vi "CRYSet Window Language.vi"(10 "sID":string) -> (1 "sMultibyte_Out":string, 2 "sID_Out":string, 3 "sUnicode_Out":string)   [LabVIEW 2013]
uses:
  CRYMainGlobal.vi
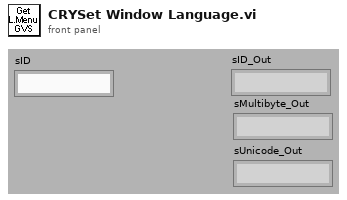
[diagram p1: front panel]
types:
  T1 = enum32{"English", "Chinese", "Korean", "Japanese", "Russian", "Chinese traditional"}
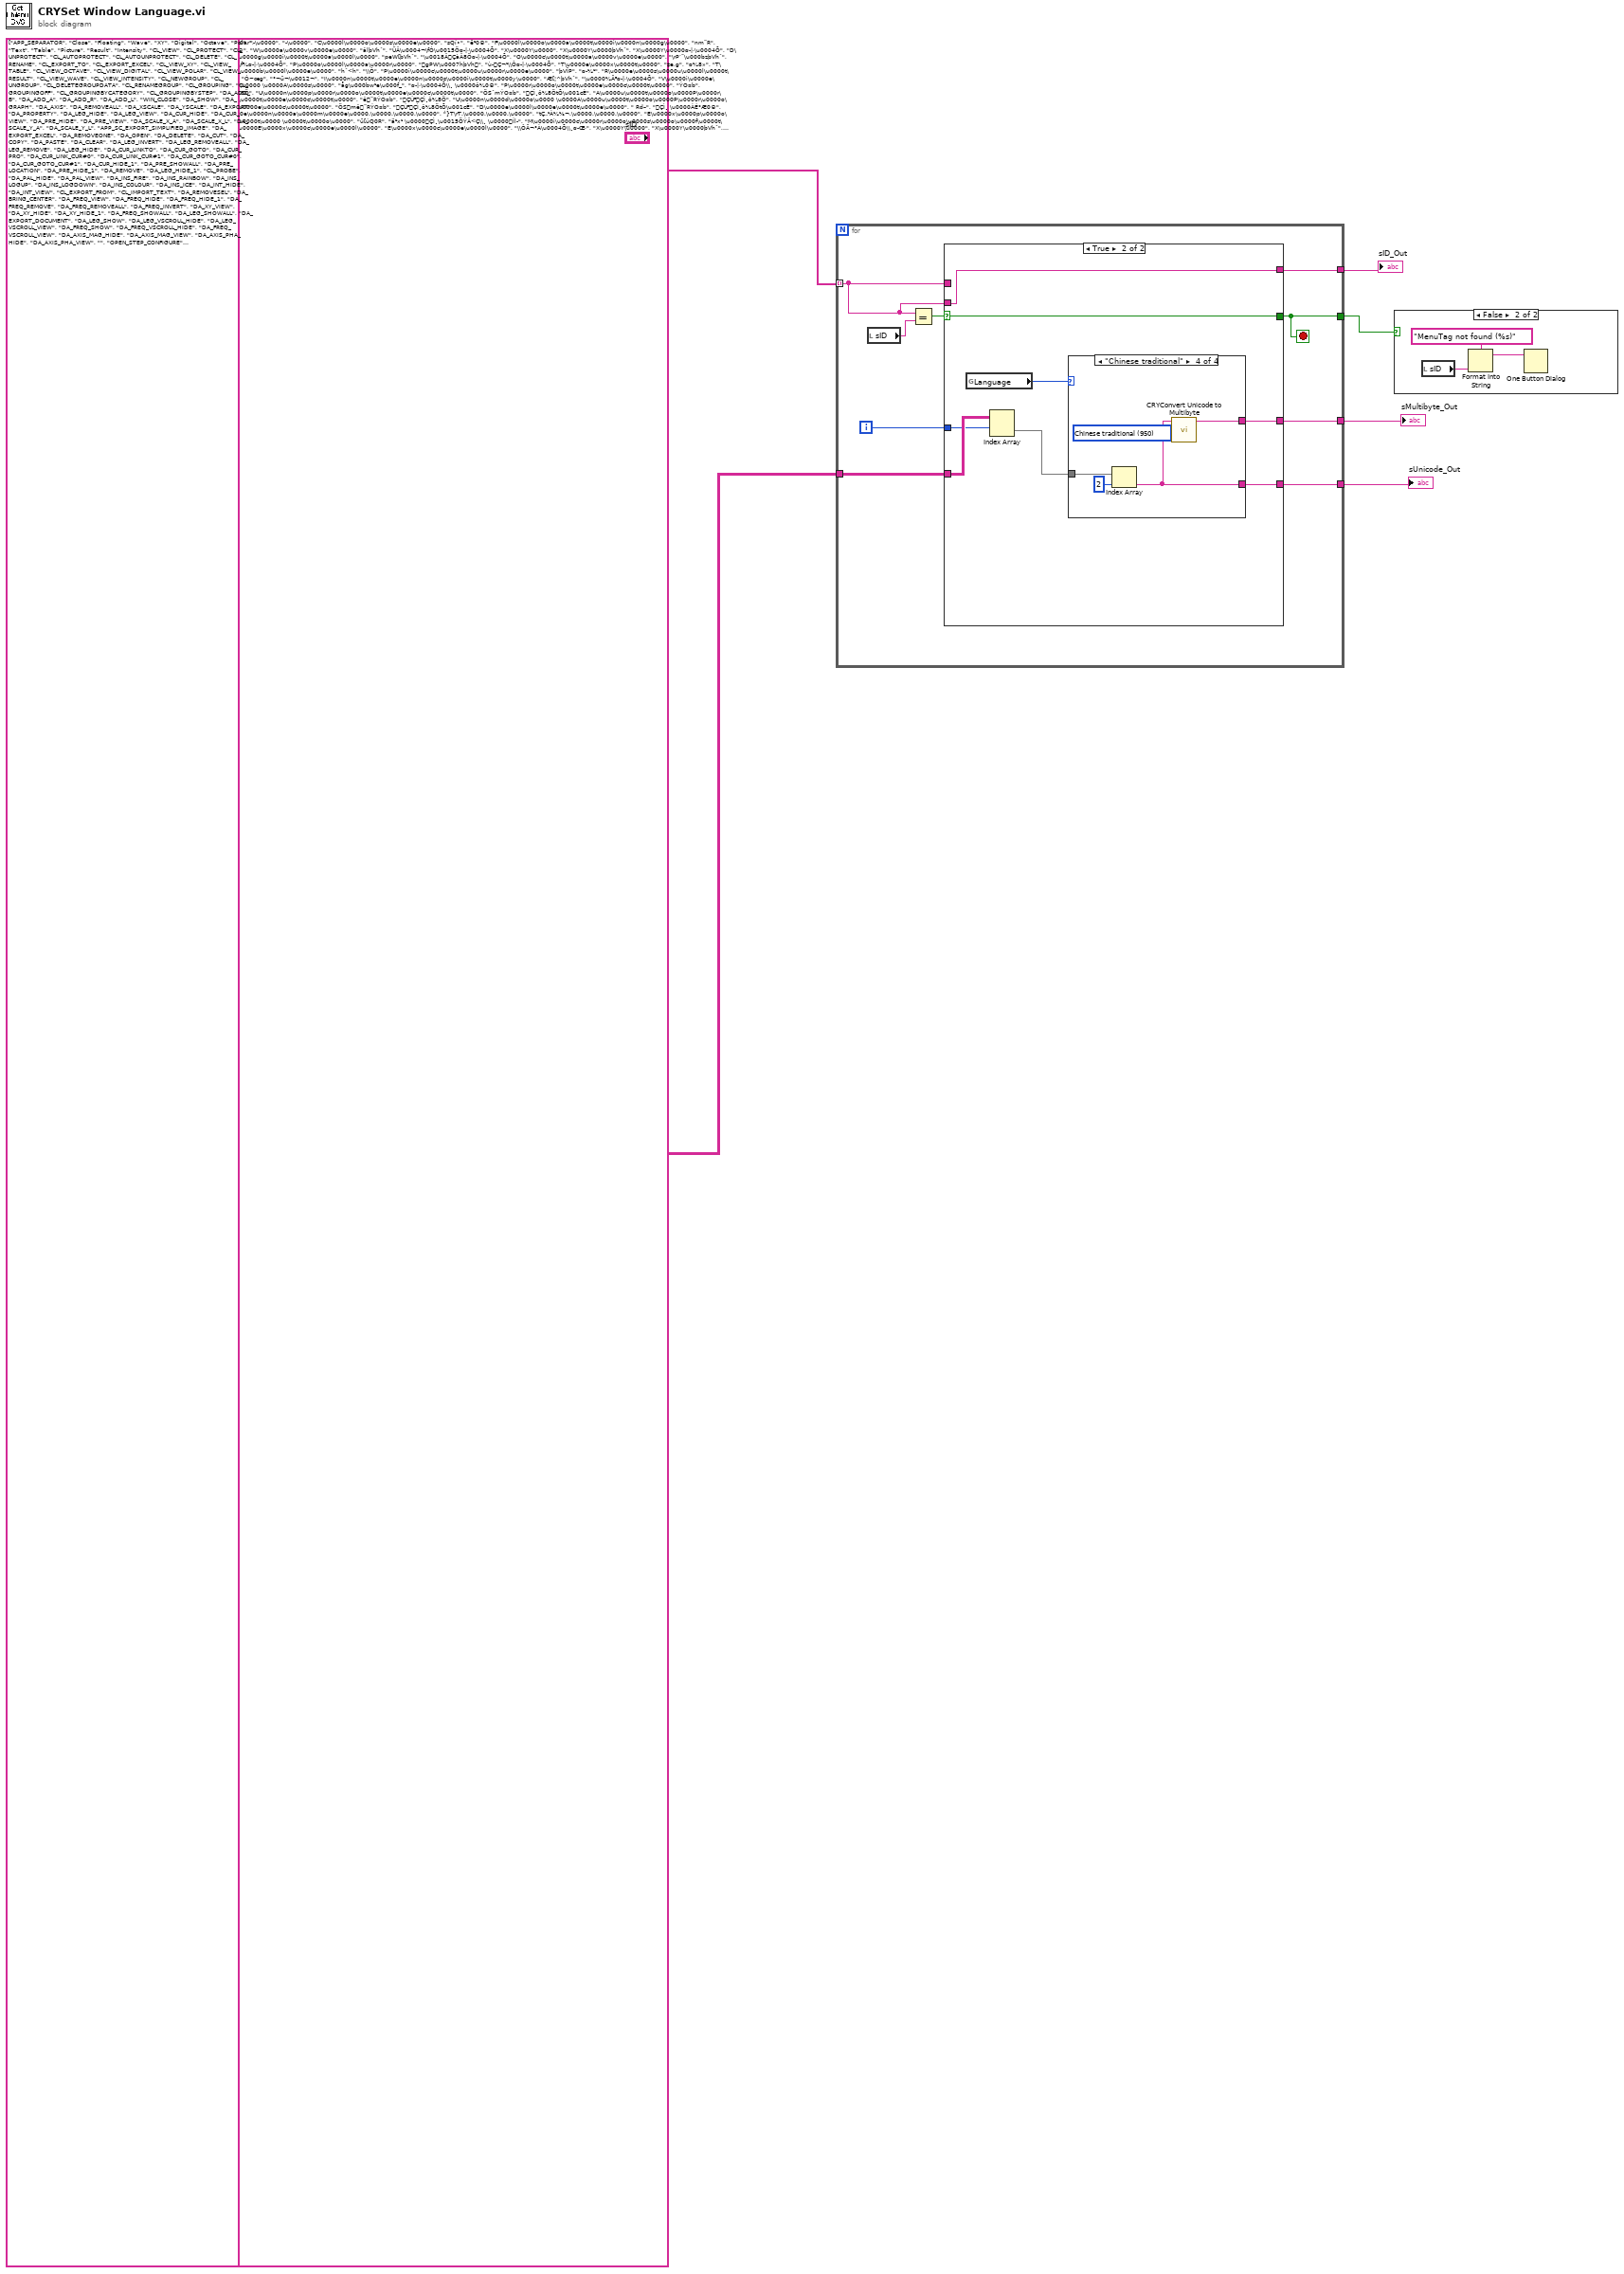
[diagram p0: block diagram]
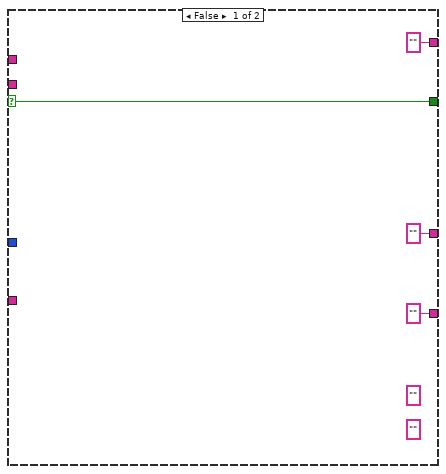
[diagram p3: hidden frame]
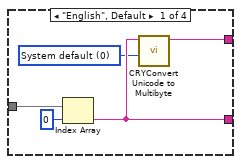
[diagram p4: hidden frame]
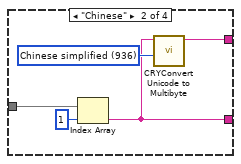
[diagram p5: hidden frame]
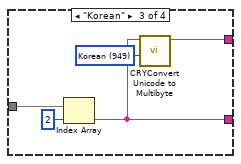
[diagram p6: hidden frame]
diagram:
  # "ASCIICODE"
  # "UNICODE"
  n1 = for {
    tunnel: string[][] [["-\u0000", "-\u0000", "-\u0000"], ["C\u0000l\u0000o\u0000s\u0000e\u0000", "sQí•", "ë²0®"], ["F\u0000l\u0000o\u0000a\u0000t\u0000i\u0000n\u0000g\u0000", "nm¨R", "D·°Æ0®"], ["W\u0000a\u0000v\u0000e\u0000", "âlþVhˆ", "ÜÂ\u0004¬\fÓ\u0015Öø­|·\u0004Õ"], ["X\u0000Y\u0000", "X\u0000Y\u0000þVhˆ", "X\u0000Y\u0000ø­|·\u0004Õ"], ["D\u0000i\u0000g\u0000i\u0000t\u0000a\u0000l\u0000", "peW[þVhˆ", "\u0018ÂÇàÂ8Öø­|·\u0004Õ"], ["O\u0000c\u0000t\u0000a\u0000v\u0000e\u0000", "\rP‘˜\u000bzþVhˆ", "%ÆÀÐ\f¾ø­|·\u0004Õ"], ["P\u0000o\u0000l\u0000a\u0000r\u0000", "gPW\u0007hþVh", "ù­Ç¬¹\\Ôø­|·\u0004Õ"], ["T\u0000e\u0000x\u0000t\u0000", "‡e,g", "ø¼8»"], ["T\u0000a\u0000b\u0000l\u0000e\u0000", "hˆ<h", "\\Ô"], ["P\u0000i\u0000c\u0000t\u0000u\u0000r\u0000e\u0000", "þVÏP", "ø­¼¹"], ["R\u0000e\u0000s\u0000u\u0000l\u0000t\u0000", "Ó~œg", "°¬ü¬\u0012¬"], ["I\u0000n\u0000t\u0000e\u0000n\u0000s\u0000i\u0000t\u0000y\u0000", "Æ[¦^þVhˆ", "\u0000¼Ä³ø­|·\u0004Õ"], ["V\u0000i\u0000e\u0000w\u0000 \u0000A\u0000s\u0000", "åg\u000bw¹e\u000f_", "ø­|·\u0004Õ\\¸ \u0000ô¼0®"], ["P\u0000r\u0000o\u0000t\u0000e\u0000c\u0000t\u0000", "ÝO¤b", "ÇÌ¸ô¼8Ö"], ["U\u0000n\u0000p\u0000r\u0000o\u0000t\u0000e\u0000c\u0000t\u0000", "ÖSˆmÝO¤b", "ÇÌ¸ô¼8ÖtÕ\u001cÈ"], ["A\u0000u\u0000t\u0000o\u0000P\u0000r\u0000o\u0000t\u0000e\u0000c\u0000t\u0000", "ê¨RÝO¤b", "ÇÙ³ÇÌ¸ô¼8Ö"], ["U\u0000n\u0000d\u0000o\u0000 \u0000A\u0000u\u0000t\u0000o\u0000P\u0000r\u0000o\u0000t\u0000e\u0000c\u0000t\u0000", "ÖSmê¨RÝO¤b", "ÇÙ³ÇÌ¸ô¼8ÖtÕ\u001cÈ"], ["D\u0000e\u0000l\u0000e\u0000t\u0000e\u0000", " Rd–", "ÇÌ¸ \u0000ÀÉ°Æ0®"], ["R\u0000e\u0000n\u0000a\u0000m\u0000e\u0000.\u0000.\u0000.\u0000", "͑}T\rT.\u0000.\u0000.\u0000", "tÇ„¹À¼½¬.\u0000.\u0000.\u0000"], ["E\u0000x\u0000p\u0000o\u0000r\u0000t\u0000 \u0000t\u0000o\u0000", "ü[úQ0R", "ä²x¹ \u0000ÇÌ¸\u0015ÖÝÂ<Ç\\¸ \u0000Íl­"], ["M\u0000i\u0000c\u0000r\u0000o\u0000s\u0000o\u0000f\u0000t\u0000 \u0000E\u0000x\u0000c\u0000e\u0000l\u0000", "E\u0000x\u0000c\u0000e\u0000l\u0000", "\\ÔÄ¬°À\u0004Õ\\¸ø­Œ·"], ["X\u0000Y\u0000", "X\u0000Y\u0000þVhˆ", "X\u0000Y\u0000ø­|·\u0004Õ"], ["T\u0000a\u0000b\u0000l\u0000e\u0000", "hˆ<h", "\\Ô=Ì8»"], ["O\u0000c\u0000t\u0000a\u0000v\u0000e\u0000", "\rP‘˜\u000bzþVhˆ", "%ÆÀÐ\f¾ø­|·\u0004Õ"], ["D\u0000i\u0000g\u0000i\u0000t\u0000a\u0000l\u0000", "peW[þVhˆ", "\u0018ÂÇàÂ8Öø­|·\u0004Õ"], ["P\u0000o\u0000l\u0000a\u0000r\u0000", "gPW\u0007hþVh", "ù­Ç¬¹\\Ôø­|·\u0004Õ"], ["R\u0000e\u0000s\u0000u\u0000l\u0000t\u0000", "Ó~œg", "°¬ü¬=Ì8»"], ["W\u0000a\u0000v\u0000e\u0000", "âlþVhˆ", "ÜÂ\u0004¬\fÓ\u0015Öø­|·\u0004Õ"], ["I\u0000n\u0000t\u0000e\u0000n\u0000s\u0000i\u0000t\u0000y\u0000", "Æ[¦^þVhˆ", "\u0000¼Ä³ø­|·\u0004Õ"], ["N\u0000e\u0000w\u0000 \u0000G\u0000r\u0000o\u0000u\u0000p\u0000", "°eú^\u0006RÄ~", "ÈÀø­ù¸"], ["U\u0000n\u0000g\u0000r\u0000o\u0000u\u0000p\u0000", "ÖSˆm\u0006RÄ~", "ø­ù¸tÕ\u001cÈ"], ["D\u0000e\u0000l\u0000e\u0000t\u0000e\u0000 \u0000G\u0000r\u0000o\u0000u\u0000p\u0000 \u0000a\u0000n\u0000d\u0000 \u0000D\u0000a\u0000t\u0000a\u0000", " Rd–\u0006RÄ~penc", "ø­ù¸ \u0000\u000f¼ \u0000ÇÌ¸ÀÉ°Æ0® \u0000"], ["R\u0000e\u0000n\u0000a\u0000m\u0000e\u0000.\u0000.\u0000.\u0000", "͑}T\rT.\u0000.\u0000.\u0000", "tÇ„¹À¼½¬.\u0000.\u0000.\u0000"], ["A\u0000u\u0000t\u0000o\u0000G\u0000r\u0000o\u0000u\u0000p\u0000i\u0000n\u0000g\u0000", "ê¨R\u0006RÄ~", "ø­ù¸TÖ"], ["A\u0000u\u0000t\u0000o\u0000G\u0000r\u0000o\u0000u\u0000p\u0000i\u0000n\u0000g\u0000 \u0000O\u0000f\u0000f\u0000", "sQíê¨R\u0006RÄ~", "ÇÙ³ø­ù¸TÖD°0®"], ["A\u0000u\u0000t\u0000o\u0000G\u0000r\u0000o\u0000u\u0000p\u0000i\u0000n\u0000g\u0000 \u0000b\u0000y\u0000 \u0000C\u0000a\u0000t\u0000e\u0000g\u0000o\u0000r\u0000y\u0000", "\tcgq{|Wê¨R\u0006RÄ~", "½X¹ÐÅ \u0000XÇ\\Õ \u0000ÇÙ³ø­ù¸TÖ"], ["A\u0000u\u0000t\u0000o\u0000G\u0000r\u0000o\u0000u\u0000p\u0000i\u0000n\u0000g\u0000 \u0000b\u0000y\u0000 \u0000S\u0000t\u0000e\u0000p\u0000", "\tcgqek¤ê¨R\u0006RÄ~", "mÕ©ºÐÅ \u0000XÇ\\Õ \u0000ÇÙ³ø­ù¸TÖ"], ["A\u0000d\u0000d\u0000 \u0000B\u0000e\u0000l\u0000o\u0000w\u0000", "\u0011T\u000bNûm R", "DÅ˜·ÐÅ \u0000½À…Ç"], ["A\u0000d\u0000d\u0000 \u0000A\u0000b\u0000o\u0000v\u0000e\u0000", "\u0011T\nNûm R", "捌信 \u0000嚼吳"], ["A\u0000d\u0000d\u0000 \u0000R\u0000i\u0000g\u0000h\u0000t\u0000", "\u0011TóSûm R", "$Æx¹½ÊÐÅ \u0000½À…Ç"], ["A\u0000d\u0000d\u0000 \u0000L\u0000e\u0000f\u0000t\u0000", "\u0011Tæ]ûm R", "|Æ½ÊÐÅ \u0000½À…Ç"], ["R\u0000e\u0000m\u0000o\u0000v\u0000e\u0000", " Rd–", "ë²0®"], ["S\u0000h\u0000o\u0000w\u0000", ">f:y", "\\ÔÜÂ"], ["G\u0000r\u0000a\u0000p\u0000h\u0000 \u0000V\u0000i\u0000e\u0000w\u0000", "ûm RþVhˆ", "ø­|·\u0004Õ \u0000”Í\u0000¬"], ["A\u0000x\u0000i\u0000s\u0000", "E^¦^/\u0000øvMO", "•Í"], ["R\u0000e\u0000m\u0000o\u0000v\u0000e\u0000 \u0000A\u0000l\u0000l\u0000", " Rd–@b\tgòf¿~", "¨ºà´ \u0000ÇÌ¸ÀÉ°Æ0®"], ["X\u0000 \u0000S\u0000c\u0000a\u0000l\u0000e\u0000", "X\u0000 \u0000\u0007h:\\", "X\u0000™ÌÄ³"], ["Y\u0000 \u0000S\u0000c\u0000a\u0000l\u0000e\u0000", "Y\u0000 \u0000\u0007h:\\", "Y\u0000™ÌÄ³"], ["E\u0000x\u0000p\u0000o\u0000r\u0000t\u0000 \u0000t\u0000o\u0000", "ü[úQ0R", "ä²x¹ \u0000ÇÌ¸\u0015ÖÝÂ<Ç\\¸ \u0000Íl­"], ["P\u0000r\u0000o\u0000p\u0000e\u0000r\u0000t\u0000i\u0000e\u0000s\u0000.\u0000.\u0000.\u0000", "^\\'`.\u0000.\u0000.\u0000", "Á1Á.\u0000.\u0000.\u0000"], ["L\u0000e\u0000g\u0000e\u0000n\u0000d\u0000", "þV‹O", "tÇ„¹©º]¸"], ["L\u0000e\u0000g\u0000e\u0000n\u0000d\u0000", "þV‹O", "tÇ„¹©º]¸"], ["C\u0000u\u0000r\u0000s\u0000o\u0000r\u0000", "8n\u0007h", " Ç\\Ô"], ["C\u0000u\u0000r\u0000s\u0000o\u0000r\u0000", "8n\u0007h", " Ç\\Ô"], ["P\u0000r\u0000e\u0000v\u0000i\u0000e\u0000w\u0000", "„˜È‰", "ø»¬¹ô¼0®"], ["P\u0000r\u0000e\u0000v\u0000i\u0000e\u0000w\u0000", "„˜È‰", "ø»¬¹ô¼0®"], ["A\u0000u\u0000t\u0000o\u0000 \u0000S\u0000c\u0000a\u0000l\u0000e\u0000", "ꁨR)>e", "ÇÙ³ÌÄ³"], ["L\u0000o\u0000g\u0000a\u0000r\u0000i\u0000t\u0000h\u0000m\u0000i\u0000c\u0000", "ù[pe", "\\¸ø­™ÌÄ³"], ["A\u0000u\u0000t\u0000o\u0000 \u0000S\u0000c\u0000a\u0000l\u0000e\u0000", "ꁨR)>e", "ÇÙ³ÌÄ³"], ["L\u0000o\u0000g\u0000a\u0000r\u0000i\u0000t\u0000h\u0000m\u0000i\u0000c\u0000", "ù[pe", "\\¸ø­™ÌÄ³"], ["S\u0000i\u0000m\u0000p\u0000l\u0000i\u0000f\u0000i\u0000e\u0000d\u0000 \u0000I\u0000m\u0000a\u0000g\u0000e\u0000", "€{\u0016S„vþVÏP", "\u0004¬è²\\Õ \u0000TÖÁÀ"], ["M\u0000i\u0000c\u0000r\u0000o\u0000s\u0000o\u0000f\u0000t\u0000 \u0000E\u0000x\u0000c\u0000e\u0000l\u0000", "E\u0000x\u0000c\u0000e\u0000l\u0000", "\\ÔÄ¬°À\u0004Õ\\¸ø­Œ·"], ["R\u0000e\u0000m\u0000o\u0000v\u0000e\u0000", " Rd–", "\\Õ\u001c¬ \u0000ÇÌ¸ÀÉ°Æ0®"], ["O\u0000p\u0000e\u0000n\u0000", "Sb\u0000_", "ôÅ0®"], ["D\u0000e\u0000l\u0000e\u0000t\u0000e\u0000", " Rd–", "ÀÉ°Æ0®"], ["C\u0000u\u0000t\u0000", "jR4", "Çt¹0®"], ["C\u0000o\u0000p\u0000y\u0000", "\rY6R", "õ¼¬À"], ["P\u0000a\u0000s\u0000t\u0000e\u0000", "4\nN", "™½tÇ0®"], ["C\u0000l\u0000e\u0000a\u0000r\u0000", "\u0005nd–", "ÀÉ°Æ0®"], ["I\u0000n\u0000v\u0000e\u0000r\u0000t\u0000", "ÍS\t", "\u0018¼\u0004È"], ["R\u0000e\u0000m\u0000o\u0000v\u0000e\u0000 \u0000A\u0000l\u0000l\u0000", " Rd–@b\tg", "¨ºà´ \u0000ÇÌ¸ÀÉ°Æ0®"], ["R\u0000e\u0000m\u0000o\u0000v\u0000e\u0000", " Rd–", "\\Õ\u001c¬ \u0000ÇÌ¸ÀÉ°Æ0®"], ["H\u0000i\u0000d\u0000e\u0000 \u0000L\u0000e\u0000g\u0000e\u0000n\u0000d\u0000", "ÏþVO", "á¬ ÁtÇ„¹ \u0000(Â0®0®"], ["L\u0000i\u0000n\u0000k\u0000 \u0000T\u0000o\u0000 \u0000P\u0000l\u0000o\u0000t\u0000", "þ”¥cØ~6R", "ø­|·\u0004ÕÐÅ \u0000(¸°¬"], ["G\u0000o\u0000 \u0000T\u0000o\u0000 \u0000C\u0000u\u0000r\u0000s\u0000o\u0000r\u0000", "l0R8n\u0007h", " Ç\\Ô\u0004ÇXÎ\\¸ \u0000.Æ0®0®"], ["C\u0000u\u0000r\u0000s\u0000o\u0000r\u0000 \u0000P\u0000r\u0000o\u0000p\u0000e\u0000r\u0000t\u0000i\u0000e\u0000s\u0000.\u0000.\u0000.\u0000", "8n\u0007h„v^\\'`.\u0000.\u0000.\u0000", " Ç\\ÔÁ1Á"], ["C\u0000u\u0000r\u0000s\u0000o\u0000r\u0000 \u00000\u0000", "8n\u0007h0\u0000", " Ç\\Ô \u00000\u0000"], ["C\u0000u\u0000r\u0000s\u0000o\u0000r\u0000 \u00001\u0000", "8n\u0007h1\u0000", " Ç\\Ô \u00001\u0000"], ["C\u0000u\u0000r\u0000s\u0000o\u0000r\u0000 \u00000\u0000", "8n\u0007h0\u0000", " Ç\\Ô \u00000\u0000"], ["C\u0000u\u0000r\u0000s\u0000o\u0000r\u0000 \u00001\u0000", "8n\u0007h1\u0000", " Ç\\Ô \u00001\u0000"], ["H\u0000i\u0000d\u0000e\u0000 \u0000C\u0000u\u0000r\u0000s\u0000o\u0000r\u0000", "Ï8n\u0007h", " Ç\\Ô(Â0®0®"], ["S\u0000h\u0000o\u0000w\u0000 \u0000A\u0000l\u0000l\u0000", ">f:y@b\tg", "\u0004È´Ìô¼ìÅüÈ0®"], ["G\u0000o\u0000 \u0000T\u0000o\u0000 \u0000L\u0000o\u0000c\u0000a\u0000t\u0000i\u0000o\u0000n\u0000", "»SMOn", "\u0004Ö¬Ç\u0004ÇXÎô¼ìÅüÈ0®"], ["H\u0000i\u0000d\u0000e\u0000 \u0000P\u0000r\u0000e\u0000v\u0000i\u0000e\u0000w\u0000", "ÏÈ", "ø»¬¹ô¼0®(Â0®0®"], ["R\u0000e\u0000m\u0000o\u0000v\u0000e\u0000", " Rd–", "ÇÌ¸ÀÉ°Æ0®"], ["H\u0000i\u0000d\u0000e\u0000 \u0000L\u0000e\u0000g\u0000e\u0000n\u0000d\u0000", "ÏÈ", "tÇ„¹©º]¸ \u0000(Â0®0®"], ["S\u0000h\u0000o\u0000w\u0000 \u0000P\u0000r\u0000o\u0000b\u0000e\u0000\u0000", ">f:y¢cˆ”", "\u0000³íÅô¼0®"], ["P\u0000a\u0000l\u0000e\u0000t\u0000t\u0000e\u0000", "þVb_å]wQ", "pÈ…È\u0010Ó"], ["P\u0000a\u0000l\u0000e\u0000t\u0000t\u0000e\u0000", "þVb_å]wQ", "pÈ…È\u0010Ó"], ["F\u0000i\u0000r\u0000e\u0000", "kp\n\u0000\u0000\u0000\n\u0000", "ˆ½8®"], ["R\u0000a\u0000i\u0000n\u0000b\u0000o\u0000w\u0000", "i_y†", "4»ÀÉ\u001c¬"], ["L\u0000o\u0000g\u0000 \u0000u\u0000p\u0000", "ù[pe\nN", "ÃÆ \u0000\\¸ø­"], ["L\u0000o\u0000g\u0000 \u0000d\u0000o\u0000w\u0000n\u0000", "ù[pe\u000bN", "DÅ˜· \u0000\\¸ø­"], ["C\u0000o\u0000l\u0000o\u0000u\u0000r\u0000", "i_r‚", "ÉÀ\b¬"], ["I\u0000c\u0000e\u0000", "°Q", "¼ÅLÇ"], ["I\u0000n\u0000t\u0000e\u0000n\u0000s\u0000i\u0000t\u0000y\u0000", "Æ[¦^þVhˆ", "\u0000¼Ä³ø­|·\u0004Õ"], ["I\u0000n\u0000t\u0000e\u0000n\u0000s\u0000i\u0000t\u0000y\u0000", "Æ[¦^þVhˆ", "\u0000¼Ä³ø­|·\u0004Õ"], ["I\u0000m\u0000p\u0000o\u0000r\u0000t\u0000 \u0000f\u0000o\u0000r\u0000m\u0000", "ÎN‡eöNü[eQ", "\fÓ|Ç\\¸€½0Ñ \u0000…Çl­"], ["T\u0000e\u0000x\u0000t\u0000 \u0000f\u0000i\u0000l\u0000e\u0000", "‡e,g‡eöN", "ø¼8»\fÓ|Ç"], ["R\u0000e\u0000m\u0000o\u0000v\u0000e\u0000 \u0000S\u0000e\u0000l\u0000e\u0000c\u0000t\u0000e\u0000d\u0000 \u0000R\u0000o\u0000w\u0000s\u0000", " Rd\t[vL", " ÁÝÐ\u001c´ \u0000ÕÇÌ¸ÀÉ°Æ0®"], ["B\u0000r\u0000i\u0000n\u0000g\u0000 \u0000t\u0000o\u0000 \u0000C\u0000e\u0000n\u0000t\u0000e\u0000r\u0000", "&^eg„v-Nô•", "\u0011ÉìÂ<Ç\\¸ \u0000tÇÙ³"], ["F\u0000r\u0000e\u0000q\u0000u\u0000e\u0000n\u0000c\u0000y\u0000", "‘˜‡s", "üÈ\fÓ\u0018Â"], ["F\u0000r\u0000e\u0000q\u0000u\u0000e\u0000n\u0000c\u0000y\u0000", "‘˜‡s", "üÈ\fÓ\u0018Â"], ["H\u0000i\u0000d\u0000e\u0000 \u0000F\u0000r\u0000e\u0000q\u0000u\u0000e\u0000n\u0000c\u0000y\u0000", "Ïs", "üÈ\fÓ\u0018Â(Â0®0®"], ["R\u0000e\u0000m\u0000o\u0000v\u0000e\u0000", " Rd–", "\\Õ\u001c¬ \u0000üÈ\fÓ\u0018ÂÀÉ°Æ0®"], ["R\u0000e\u0000m\u0000o\u0000v\u0000e\u0000 \u0000A\u0000l\u0000l\u0000", " Rd–@b\tg", "¨ºà´ \u0000üÈ\fÓ\u0018ÂÀÉ°Æ0®"], ["I\u0000n\u0000v\u0000e\u0000r\u0000t\u0000", "\u0012Pn", "\u0018¼\u0004È"], ["X\u0000Y\u0000 \u0000G\u0000r\u0000a\u0000p\u0000h\u0000", "X\u0000Y\u0000þVhˆ", "X\u0000Y\u0000ø­|·\u0004Õ"], ["X\u0000Y\u0000 \u0000G\u0000r\u0000a\u0000p\u0000h\u0000", "X\u0000Y\u0000þVhˆ", "X\u0000Y\u0000ø­|·\u0004Õ"], ["H\u0000i\u0000d\u0000e\u0000 \u0000X\u0000Y\u0000 \u0000G\u0000r\u0000a\u0000p\u0000h\u0000", "ÏX\u0000Y\u0000þVh", "X\u0000Y\u0000ø­|·\u0004Õ \u0000(Â0®0®"], ["S\u0000h\u0000o\u0000w\u0000 \u0000A\u0000l\u0000l\u0000", ">f:y@b\tg‘˜‡s", "¨ºà´ \u0000 \u0000üÈ\fÓ\u0018Âô¼ìÅüÈ0®"], ["S\u0000h\u0000o\u0000w\u0000 \u0000A\u0000l\u0000l\u0000", ">f:y@b\tg", "¨ºà´ \u0000 \u0000ÇÌ¸ô¼ìÅüÈ0®"], ["D\u0000o\u0000c\u0000u\u0000m\u0000e\u0000n\u0000t\u0000", "‡e,g", "8»\u001cÁ¸ÓÑÉ=Ì8»"], ["S\u0000h\u0000o\u0000w\u0000", ">f:y", "\\ÔÜÂ"], ["V\u0000e\u0000r\u0000t\u0000i\u0000c\u0000a\u0000l\u0000 \u0000S\u0000c\u0000r\u0000o\u0000l\u0000l\u0000b\u0000a\u0000r\u0000", "‚WôvÚn¨Rag", "\u0018ÂÁÉtÇÙ³`·"], ["V\u0000e\u0000r\u0000t\u0000i\u0000c\u0000a\u0000l\u0000 \u0000S\u0000c\u0000r\u0000o\u0000l\u0000l\u0000b\u0000a\u0000r\u0000", "‚WôvÚn¨Rag", "\u0018ÂÁÉtÇÙ³`·"], ["S\u0000h\u0000o\u0000w\u0000", ">f:y", "\\ÔÜÂ"], ["V\u0000e\u0000r\u0000t\u0000i\u0000c\u0000a\u0000l\u0000 \u0000S\u0000c\u0000r\u0000o\u0000l\u0000l\u0000b\u0000a\u0000r\u0000", "‚WôvÚn¨Rag", "\u0018ÂÁÉtÇÙ³`·"], ["V\u0000e\u0000r\u0000t\u0000i\u0000c\u0000a\u0000l\u0000 \u0000S\u0000c\u0000r\u0000o\u0000l\u0000l\u0000b\u0000a\u0000r\u0000", "‚WôvÚn¨Rag", "\u0018ÂÁÉtÇÙ³`·"], ["M\u0000a\u0000g\u0000n\u0000i\u0000t\u0000u\u0000d\u0000e\u0000", "E^¦^", "ÄÉíÓ"], ["M\u0000a\u0000g\u0000n\u0000i\u0000t\u0000u\u0000d\u0000e\u0000", "E^¦^", "ÄÉíÓ"], ["P\u0000h\u0000a\u0000s\u0000e\u0000", "øvMO", "\u0004ÇÁÀ"], ["P\u0000h\u0000a\u0000s\u0000e\u0000", "øvMO", "\u0004ÇÁÀ"], ["", "", ""], ["C\u0000o\u0000n\u0000f\u0000i\u0000g\u0000u\u0000r\u0000e\u0000 \u0000S\u0000t\u0000e\u0000p\u0000.\u0000.\u0000.\u0000", "ek¤šÓ~„g.\u0000.\u0000.\u0000", "¸ÓÑÉ0®l­1Á.\u0000.\u0000.\u0000"], ["M\u0000o\u0000v\u0000e\u0000 \u0000D\u0000o\u0000w\u0000n\u0000", "\u0011T\u000bN\n\u0000\u0000\u0000", "DÅ˜·\\¸ \u0000tÇÙ³"], ["M\u0000o\u0000v\u0000e\u0000 \u0000U\u0000p\u0000", "\u0011T\nN", "°Æ\\¸ \u0000tÇÙ³"], ["D\u0000e\u0000l\u0000e\u0000t\u0000e\u0000", " Rd–", "­À\u001cÈ"], ["C\u0000o\u0000n\u0000f\u0000i\u0000g\u0000u\u0000r\u0000e\u0000 \u0000S\u0000e\u0000q\u0000u\u0000e\u0000n\u0000c\u0000e\u0000.\u0000.\u0000.\u0000", "^\u0017RÓ~g.\u0000.\u0000.\u0000", "ü¬\u001cÈ,¸l­1Á.\u0000.\u0000.\u0000"], ["R\u0000e\u0000n\u0000a\u0000m\u0000e\u0000.\u0000.\u0000.\u0000", "͑}T\rT.\u0000.\u0000.\u0000", "tÇ„¹À¼½¬.\u0000.\u0000.\u0000"], ["", "", ""], ["N\u0000e\u0000w\u0000.\u0000.\u0000.\u0000", "°eú^.\u0000.\u0000.\u0000", "ÈÀmÕ©º.\u0000.\u0000.\u0000"]] -> [w14]
    tunnel: [w12] -> w6
    tunnel: [w11] -> w5
    tunnel: string[] ["APP_SEPARATOR", "Close", "Floating", "Wave", "XY", "Digital", "Octave", "Polar", "Text", "Table", "Picture", "Result", "Intensity", "CL_VIEW", "CL_PROTECT", "CL_UNPROTECT", "CL_AUTOPROTECT", "CL_AUTOUNPROTECT", "CL_DELETE", "CL_RENAME", "CL_EXPORT_TO", "CL_EXPORT_EXCEL", "CL_VIEW_XY", "CL_VIEW_TABLE", "CL_VIEW_OCTAVE", "CL_VIEW_DIGITAL", "CL_VIEW_POLAR", "CL_VIEW_RESULT", "CL_VIEW_WAVE", "CL_VIEW_INTENSITY", "CL_NEWGROUP", "CL_UNGROUP", "CL_DELETEGROUPDATA", "CL_RENAMEGROUP", "CL_GROUPING", "CL_GROUPINGOFF", "CL_GROUPINGBYCATEGORY", "CL_GROUPINGBYSTEP", "DA_ADD_B", "DA_ADD_A", "DA_ADD_R", "DA_ADD_L", "WIN_CLOSE", "DA_SHOW", "DA_GRAPH", "DA_AXIS", "DA_REMOVEALL", "DA_XSCALE", "DA_YSCALE", "DA_EXPORT", "DA_PROPERTY", "DA_LEG_HIDE", "DA_LEG_VIEW", "DA_CUR_HIDE", "DA_CUR_VIEW", "DA_PRE_HIDE", "DA_PRE_VIEW", "DA_SCALE_X_A", "DA_SCALE_X_L", "DA_SCALE_Y_A", "DA_SCALE_Y_L", "APP_SC_EXPORT_SIMPLIFIED_IMAGE", "DA_EXPORT_EXCEL", "DA_REMOVEONE", "DA_OPEN", "DA_DELETE", "DA_CUT", "DA_COPY", "DA_PASTE", "DA_CLEAR", "DA_LEG_INVERT", "DA_LEG_REMOVEALL", "DA_LEG_REMOVE", "DA_LEG_HIDE", "DA_CUR_LINKTO", "DA_CUR_GOTO", "DA_CUR_PRO", "DA_CUR_LINK_CUR#0", "DA_CUR_LINK_CUR#1", "DA_CUR_GOTO_CUR#0", "DA_CUR_GOTO_CUR#1", "DA_CUR_HIDE_1", "DA_PRE_SHOWALL", "DA_PRE_LOCATION", "DA_PRE_HIDE_1", "DA_REMOVE", "DA_LEG_HIDE_1", "CL_PROBE", "DA_PAL_HIDE", "DA_PAL_VIEW", "DA_INS_FIRE", "DA_INS_RAINBOW", "DA_INS_LOGUP", "DA_INS_LOGDOWN", "DA_INS_COLOUR", "DA_INS_ICE", "DA_INT_HIDE", "DA_INT_VIEW", "CL_EXPORT_FROM", "CL_IMPORT_TEXT", "DA_REMOVESEL", "DA_BRING_CENTER", "DA_FREQ_VIEW", "DA_FREQ_HIDE", "DA_FREQ_HIDE_1", "DA_FREQ_REMOVE", "DA_FREQ_REMOVEALL", "DA_FREQ_INVERT", "DA_XY_VIEW", "DA_XY_HIDE", "DA_XY_HIDE_1", "DA_FREQ_SHOWALL", "DA_LEG_SHOWALL", "DA_EXPORT_DOCUMENT", "DA_LEG_SHOW", "DA_LEG_VSCROLL_HIDE", "DA_LEG_VSCROLL_VIEW", "DA_FREQ_SHOW", "DA_FREQ_VSCROLL_HIDE", "DA_FREQ_VSCROLL_VIEW", "DA_AXIS_MAG_HIDE", "DA_AXIS_MAG_VIEW", "DA_AXIS_PHA_HIDE", "DA_AXIS_PHA_VIEW", "", "OPEN_STEP_CONFIGURE", "STEP_MOVE_DOWN", "STEP_MOVE_UP", "STEP_DELETE", "OPEN_SEQUENCE_CONFIGURE", "STEP_RENAME", "", "AD_NEW"] -> [w7] mode=indexing
    tunnel: [w9] -> w4
    tunnel: [w8] -> w3
    i -> [w10]
    stop <- w8 stop-if-true
    n2 = local read "sID"() -> (w15:string)
    n3 = Equal?(x=w7, y=w15) -> (x = y?=w13:bool)
    n4 = case shown="True" w13 {
      selector: w13 -> [w17 w25]
      tunnel: w14 -> [_ w24]
      tunnel: ["" ("Multibyte string") w27] -> w12
      tunnel: ["" w26] -> w11
      tunnel: [w17 w25] -> w8
      tunnel: w10 -> [_ w23]
      tunnel: w7 -> [_ _]
      tunnel: w7 -> [_ w21]
      tunnel: ["" w21] -> w9
      frame False {
        (unwired) ""
        (unwired) ""
      }
      frame True {
        n5 = global read "CRYMainGlobal.vi" "Language"() -> (w20:T1)
        n6 = Index Array(array=w24, index (row)=w23) -> (element=w22:string[])  [unwired: 1 in]
        n7 = case shown="\"Chinese traditional\"" w20 {
          tunnel: w22 -> [w32 w35 w39 w44]
          tunnel: [w30 w33 w40 w45] -> w26
          tunnel: [w28 w34 w41 w46] -> w27
          frame "English", Default {
            w29 = 0 items=["System default"=0, "Latin-1"=1252, "Japanese"=932, "Korean"=947, "Chinese simplified"=936, "Chinese traditional"=950, "Central Europe"=1250, "Cyrillic"=1251, "Greek"=1253, "Turkish"=1254, "Hebrew"=1255, "Arabic"=1256, "Baltic"=1257, "Thai"=874, "Vietnamese"=783, "UTF8"=65001, "UTF-7"=65000] ("Code Page")
            n8 = Index Array(array=w32, index=0) -> (element=w30:string)
            n9 = call "CRYConvert Unicode to Multibyte.vi"("Code Page"=w29, "Unicode String"=w30) -> ("Multibyte string"=w28:string)  [unwired: 8 in, 1 out]
          }
          frame "Chinese" {
            w36 = 936 items=["System default"=0, "Latin-1"=1252, "Japanese"=932, "Korean"=947, "Chinese simplified"=936, "Chinese traditional"=950, "Central Europe"=1250, "Cyrillic"=1251, "Greek"=1253, "Turkish"=1254, "Hebrew"=1255, "Arabic"=1256, "Baltic"=1257, "Thai"=874, "Vietnamese"=783, "UTF8"=65001, "UTF-7"=65000] ("Code Page")
            n10 = Index Array(array=w35, index=1) -> (element=w33:string)
            n11 = call "CRYConvert Unicode to Multibyte.vi"("Code Page"=w36, "Unicode String"=w33) -> ("Multibyte string"=w34:string)  [unwired: 8 in, 1 out]
          }
          frame "Korean" {
            w38 = 949 items=["System default"=0, "Latin-1"=1252, "Japanese"=932, "Korean"=949, "Chinese simplified"=936, "Chinese traditional"=950, "Central Europe"=1250, "Cyrillic"=1251, "Greek"=1253, "Turkish"=1254, "Hebrew"=1255, "Arabic"=1256, "Baltic"=1257, "Thai"=874, "Vietnamese"=783, "UTF8"=65001, "UTF-7"=65000] ("Code Page")
            n12 = Index Array(array=w39, index=2) -> (element=w40:string)
            n13 = call "CRYConvert Unicode to Multibyte.vi"("Code Page"=w38, "Unicode String"=w40) -> ("Multibyte string"=w41:string)  [unwired: 8 in, 1 out]
          }
          frame "Chinese traditional" {
            w43 = 950 items=["System default"=0, "Latin-1"=1252, "Japanese"=932, "Korean"=949, "Chinese simplified"=936, "Chinese traditional"=950, "Central Europe"=1250, "Cyrillic"=1251, "Greek"=1253, "Turkish"=1254, "Hebrew"=1255, "Arabic"=1256, "Baltic"=1257, "Thai"=874, "Vietnamese"=783, "UTF8"=65001, "UTF-7"=65000] ("Code Page")
            n14 = Index Array(array=w44, index=2) -> (element=w45:string)
            n15 = call "CRYConvert Unicode to Multibyte.vi"("Code Page"=w43, "Unicode String"=w45) -> ("Multibyte string"=w46:string)  [unwired: 8 in, 1 out]
          }
        }
      }
    }
  }
  "sMultibyte_Out" <- w6
  "sUnicode_Out" <- w5
  "sID_Out" <- w4
  n16 = case shown="False" w3 {
    frame True {
    }
    frame False {
      n17 = local read "sID"() -> (w49:string)
      n18 = Format Into String(format string="MenuTag not found (%s)", w49) -> (resulting string=w48:string)  [unwired: 2 in, 1 out]
      n19 = One Button Dialog(message=w48) -> ()  [unwired: 1 in, 1 out]
    }
  }
